vi "Pracownia_6_maska.vi"() -> ()   [LabVIEW 2023]
uses:
  Pracownia_6_global.vi
panel:
  out "Array 2":bool[](array[boolean])
  in  "Array":bool[](array[boolean])
  out "Tablica Bitów":bool[](array[boolean])
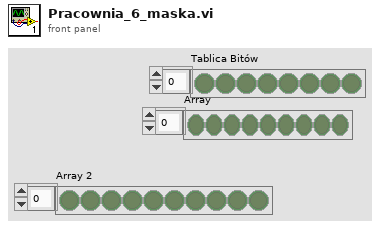
[diagram p1: front panel]
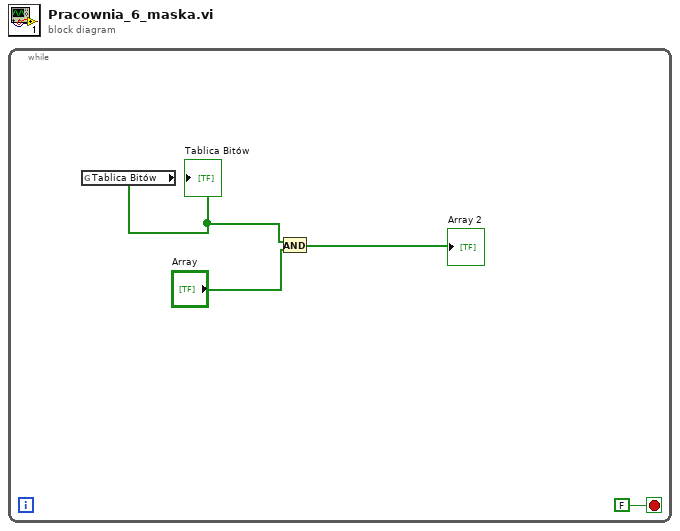
[diagram p0: block diagram]
diagram:
  n1 = while {
    stop <- FALSE stop-if-true
    n2 = global read "Pracownia_6_global.vi" "Tablica Bitów"() -> (w4:bool[])
    "Tablica Bitów" <- w4
    n3 = And(x=w4, y="Array") -> (x .and. y?=→"Array 2":bool[])
  }
